vi "Group Name.vi"(8 "error in (no error)":errorcluster, 11 "Group Buffer DBL in":refnum<class "Group Buffer DBL.lvclass">) -> (0 "error out":errorcluster, 2 "Name":string, 3 "Group Buffer DBL out":refnum<class "Group Buffer DBL.lvclass">)   [LabVIEW 2020, in "VolatusHistorian.lvlib" / "Group Buffer DBL.lvclass"]
uses:
  Group Buffer DBL.lvclass
  Group Buffer DBL.lvclass/Group Buffer DBL.ctl
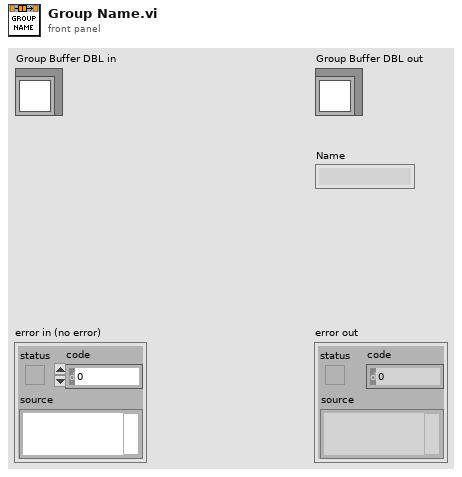
[diagram p1: front panel]
types:
  T1 = typedef "VolatusHistorian.lvlib/Group Buffer DBL.lvclass/Ref.ctl" = cluster{"Time":refnum<queue>, "Channel Name Map":map{string, i32}, "Group Info":T2, "Channels":refnum<class "Channel Buffer DBL.lvclass">[], "Channel Names":string[]}
  T2 = typedef "VectoConfig.lvlib/Group Info.ctl" = cluster{"System":string, "Cluster":string, "Node":string, "Task":string, "Name":string}
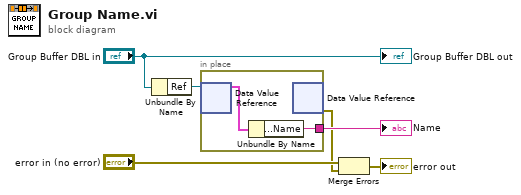
[diagram p0: block diagram]
diagram:
  n1 = Unbundle By Name("Group Buffer DBL in") -> ("Ref"=w5:refnum<data-value>)
  n2 = in-place {
    in-place-border: [w7] -> w3
    n3 = in-place-dvr #1(w5) -> (w8:T1)  [unwired: 1 out]
    n4 = Unbundle By Name(w8) -> ("Group Info.Name"=w7:string)
    n5 = in-place-dvr #1() -> (w1:errorcluster)  [unwired: 1 in, 1 out]
  }
  "Name" <- w3
  n6 = Merge Errors("error in (no error)", w1) -> (→"error out":errorcluster)
  "Group Buffer DBL out" <- "Group Buffer DBL in"
